vi "Test Morphology Stuctured Element.vi"(8 "error in (no error)":errorcluster, 11 "Test Case In":refnum<class "Image.lvclass">) -> (0 "error out":errorcluster, 3 "Test Case Out":refnum<class "Image.lvclass">)   [LabVIEW 2020, in "g_ar_toolkit.test.lvlib" / "Image.lvclass"]
uses:
  Image.lvclass
  C:/Program Files (x86)/National Instruments/LabVIEW 2020/vi.lib/Astemes/LUnit/Test Case.lvclass
  g_ar_toolkit.common/Image Size (Integer).ctl
  g_ar_toolkit.common/Image Point (Integer).ctl
  <vilib>/Astemes/LUnit/Test Case.lvclass/Test Case.ctl
  9b413f91-239b-4912-afd1-70c67bce71f4.vi
  g_ar_toolkit.image/Get Morphology Structuring Element (Rectangle).vi
  g_ar_toolkit.image/Get Morphology Structuring Element (Elipse).vi
  g_ar_toolkit.image/Get Morphology Structuring Element (Cross).vi
  4993e8ee-a06a-463a-9684-69129f64d5ce.vi
  g_ar_toolkit.image/MorphStructuringElementCore.vi
  <vilib>/Astemes/LUnit/Append Pass Result.vi
  <vilib>/Astemes/LUnit/Append Fail Result.vi
  <vilib>/Astemes/LUnit/Describe Comparison.vi
  4993e8ee-a06a-463a-9684-69129f64d5ce.vi/9c5d11cd-9439-4240-a1ee-d9baace9c924.vi
  <vilib>/Astemes/LUnit/Run In UI.vi
  <vilib>/Utility/error.llb/Clear Errors.vi
  g_ar_toolkit.common/Module Path.vi
  <vilib>/Utility/error.llb/Error Cluster From Error Code.vi
  <vilib>/Astemes/LUnit/Describe Variant.vi
  g_ar_toolkit.image/g_ar_toolkit.image.lvlib
  g_ar_toolkit.common/g_ar_toolkit.common.lvlib
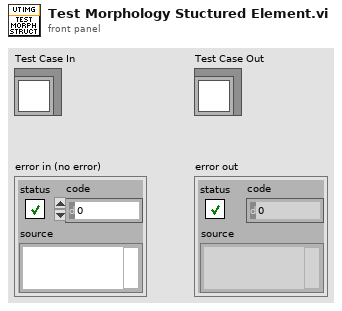
[diagram p1: front panel]
types:
  T1 = typedef "g_ar_toolkit.common.lvlib/Image Size (Integer).ctl" = cluster{"Width":u16, "Height":u16}
  T2 = typedef "g_ar_toolkit.common.lvlib/Image Point (Integer).ctl" = cluster{"x":i32, "y":i32}
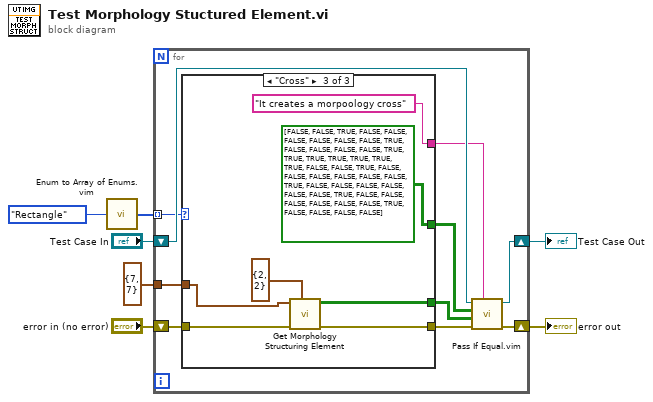
[diagram p0: block diagram]
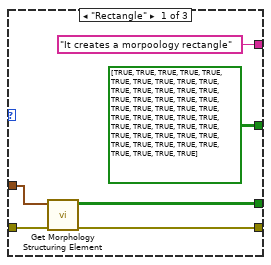
[diagram p2: hidden frame]
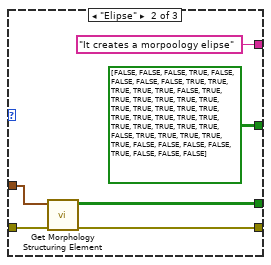
[diagram p3: hidden frame]
diagram:
  n1 = call "Enum to Array of Enums.vim"("enum"=enum16{"Rectangle", "Cross", "Elipse"}."Rectangle") -> ("array of enums"=w1:enum16{"Rectangle", "Cross", "Elipse"}[])
  n2 = for {
    tunnel: T1 {"Width"=7, "Height"=7} ("Size") -> [w14]
    shift-right: [w16] -> w6
    shift-left: "Test Case In" -> [w17]
    shift-right: [w15] -> w5
    shift-left: "error in (no error)" -> [w13]
    tunnel: w1 -> [w8] mode=indexing
    n3 = case shown="\"Cross\"" w8 {
      tunnel: w14 -> [w23 w29 w36]
      tunnel: w13 -> [w22 w28 w35]
      tunnel: [w21 w27 w34] -> w12
      tunnel: [bool[][] [[TRUE, TRUE, TRUE, TRUE, TRUE, TRUE, TRUE], [TRUE, TRUE, TRUE, TRUE, TRUE, TRUE, TRUE], [TRUE, TRUE, TRUE, TRUE, TRUE, TRUE, TRUE], [TRUE, TRUE, TRUE, TRUE, TRUE, TRUE, TRUE], [TRUE, TRUE, TRUE, TRUE, TRUE, TRUE, TRUE], [TRUE, TRUE, TRUE, TRUE, TRUE, TRUE, TRUE], [TRUE, TRUE, TRUE, TRUE, TRUE, TRUE, TRUE]] ("Structuring Element") bool[][] [[FALSE, FALSE, FALSE, TRUE, FALSE, FALSE, FALSE], [FALSE, TRUE, TRUE, TRUE, TRUE, TRUE, FALSE], [TRUE, TRUE, TRUE, TRUE, TRUE, TRUE, TRUE], [TRUE, TRUE, TRUE, TRUE, TRUE, TRUE, TRUE], [TRUE, TRUE, TRUE, TRUE, TRUE, TRUE, TRUE], [FALSE, TRUE, TRUE, TRUE, TRUE, TRUE, FALSE], [FALSE, FALSE, FALSE, TRUE, FALSE, FALSE, FALSE]] ("Structuring Element 3") bool[][] [[FALSE, FALSE, TRUE, FALSE, FALSE, FALSE, FALSE], [FALSE, FALSE, TRUE, FALSE, FALSE, FALSE, FALSE], [TRUE, TRUE, TRUE, TRUE, TRUE, TRUE, TRUE], [FALSE, FALSE, TRUE, FALSE, FALSE, FALSE, FALSE], [FALSE, FALSE, TRUE, FALSE, FALSE, FALSE, FALSE], [FALSE, FALSE, TRUE, FALSE, FALSE, FALSE, FALSE], [FALSE, FALSE, TRUE, FALSE, FALSE, FALSE, FALSE]] ("Structuring Element 2")] -> w11
      tunnel: [w19 w26 w33] -> w10
      tunnel: ["It creates a morpoology rectangle" ("Description") "It creates a morpoology elipse" ("Description") "It creates a morpoology cross" ("Description")] -> w9
      frame "Rectangle" {
        n4 = call-poly "Get Morphology Structuring Element.vi"("error in (no error)"=w22, "Size"=w23) -> ("error out"=w21:errorcluster, "Structuring Element"=w19:bool[][])  [unwired: 8 in]
      }
      frame "Elipse" {
        n5 = call-poly "Get Morphology Structuring Element.vi"("error in (no error)"=w28, "Size"=w29) -> ("error out"=w27:errorcluster, "Structuring Element"=w26:bool[][])  [unwired: 8 in]
      }
      frame "Cross" {
        n6 = call-poly "Get Morphology Structuring Element.vi"("Anchor (Default: -1, -1 Use Centre)"=T2 {"x"=2, "y"=2}, "error in (no error)"=w35, "Size"=w36) -> ("error out"=w34:errorcluster, "Structuring Element"=w33:bool[][])  [unwired: 7 in]
      }
    }
    n7 = call "Pass If Equal.vim"("Description"=w9, "error in (no error)"=w12, "Actual"=w10, "Expected"=w11, "LUnit Test Case In"=w17) -> ("error out"=w15:errorcluster, "LUnit Test Case Out"=w16:refnum<class "Image.lvclass">)  [unwired: 5 in]
  }
  "error out" <- w5
  "Test Case Out" <- w6
